vi "Change Camera.vi"(8 "error in (no error)":errorcluster, 10 "New Camera":string, 11 "IMAQdx Actor in":refnum<class "IMAQdx Actor.lvclass">) -> (0 "error out":errorcluster, 3 "IMAQdx Actor out":refnum<class "IMAQdx Actor.lvclass">)   [LabVIEW 2014, in "IMAQdx Actor.lvlib" / "IMAQdx Actor.lvclass"]
uses:
  IMAQdx Actor.lvclass
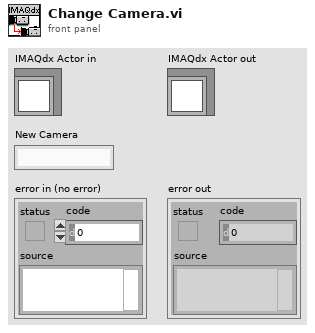
[diagram p1: front panel]
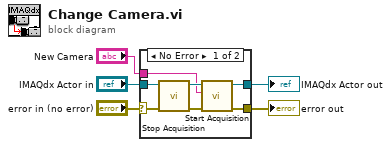
[diagram p0: block diagram]
diagram:
  n1 = case shown="No Error" "error in (no error)" {
    selector: "error in (no error)" -> [w6 w13]
    tunnel: "IMAQdx Actor in" -> [w11 w14]
    tunnel: "New Camera" -> [w9 _]
    tunnel: [w8 w14] -> w3
    tunnel: [w7 w13] -> w2
    frame No Error {
      n2 = call-dynamic "Stop Acquisition.vi"("error in (no error)"=w6, "IMAQdx Actor in"=w11) -> ("error out"=w10:errorcluster, "IMAQdx Actor out"=w12:refnum<class "IMAQdx Actor.lvclass">)  [unwired: 8 in]
      n3 = call-dynamic "Start Acquisition.vi"("error in (no error)"=w10, "Camera Name"=w9, "IMAQdx Actor in"=w12) -> ("error out"=w7:errorcluster, "IMAQdx Actor out"=w8:refnum<class "IMAQdx Actor.lvclass">)  [unwired: 7 in]
    }
    frame Error {
    }
  }
  "error out" <- w2
  "IMAQdx Actor out" <- w3
